vi "SNTP Light RT Driver VI.vi"(6 "Device Clock":string, 9 "Device Inputs FIFO":refnum<k33>, 10 "Device Outputs FIFO":refnum<k33>, 11 "Device Reference":T1 format="%.0x") -> ()   [LabVIEW 2013, in "SNTP Light Custom Device Engine.lvlib"]
uses:
  SNTP Light Custom Device Engine.lvlib
  <vilib>/NI Veristand/Custom Device API/Custom Device Item Ref.ctl
  <vilib>/NI Veristand/Custom Device API/Custom Device Channel Type.ctl
  RT_Configuration_Data.ctl
  <vilib>/NI Veristand/Custom Device API/Custom Device Timed Loop Priority.ctl
  <vilib>/Platform/TimedLoop/XDataNode/timing_clust.ctl
  <vilib>/Platform/TimedLoop/XDataNode/nitl_modes.ctl
  <vilib>/Platform/TimedLoop/XDataNode/wakeup.ctl
  <userlib>/_OpenG.lib/error/error.llb/Filter Error Codes (Array)__ogtk.vi
  <vilib>/NI Veristand/Custom Device API/Get Item Property (String).vi
  <vilib>/NI Veristand/Custom Device API/Get Item Property (U16).vi
  <vilib>/NI Veristand/Custom Device API/Get Item Property (Double).vi
  <vilib>/NI Veristand/Custom Device API/Get Item Property (Boolean).vi
  RT Driver_Global.vi
  <vilib>/platform/TimedLoop/XDataNode/XDataNode.xnode
  <vilib>/NI Veristand/Custom Device API/Custom Device API.lvlib
  <vilib>/NI Veristand/Custom Device Tools/Custom Device Utility Library/Custom Device Utility Library.lvlib
  <vilib>/NI_Real-Time Target Support.lvlib
  <vilib>/nisyscfg/nisyscfg.lvlib
  <vilib>/Platform/TimedLoop/XDataNode/XDNodeRunTimeDep.lvlib
panel:
  in  "stop":bool
  in  "Initialization Status Notifier":refnum<notifier>
  in  "Status Notifier":refnum<notifier>
  # "Custom Device Template\nv1.0"
  # "Use this template as a starting point for creating a custom device code module. The input controls shown here are specially named controls that the system will use to provide the device loop with data. The controls are not required for the device loop to run. For instance, if the device doesn't produce any output data, then you don't need the Device Outputs FIFO control. If you do use these controls, however, they need to have these exact names to be functional."
  # "The optional status notifier element is used to notify the RT engine of the last state of the custom device, and to indicate the device has completed execution. If this control is not used, a default No Error value is returned to the system when the device finishes execution.\n\nNote: This error state is not checked until the system shuts down. Use an output status channel to send more immediate status values to the system."
  # "This optional input can be used to send the VeriStand Engine the final status of the custom device initalization process. If this control exists on the custom device front panel, the VeriStand Engine will wait for a status update before starting up. If the custom device reports an error, that will abort the execution of the current configuration in the VeriStand Engine.\n\nThis control can be deleted if the custom device does not need to send the initialization status update."
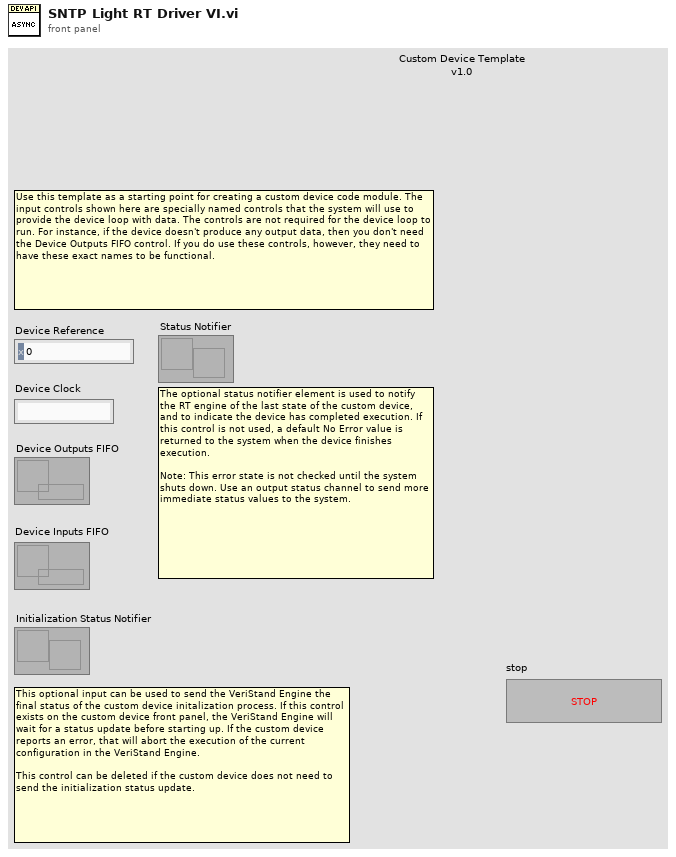
[diagram p1: front panel]
types:
  T1 = typedef "Custom Device API.lvlib/Custom Device Item Ref.ctl" = u64
  T2 = typedef "SNTP Light Custom Device Engine.lvlib/RT_Configuration_Data.ctl" = cluster{"Server IP Address":string, "UDP Port":u16, "Synchronization Interval":dbl, "Synchronization Threshold":dbl, "Debug Output Strings":bool, "Maximum Offset To Apply":dbl}
  T3 = typedef "Custom Device API.lvlib/Custom Device Channel Type.ctl" = enum16{"Input", "Output"}
  T4 = typedef "Custom Device API.lvlib/Custom Device Timed Loop Priority.ctl" = enum32{"Low", "Medium", "High"}
  T5 = typedef "XDNodeRunTimeDep.lvlib/timing_clust.ctl" = cluster{"Expected End [f-1]":u64, "Actual End [f-1]":u64, "Finished Late? [f-1]":bool, "Expected End [i-1]":u64, "Actual End [i-1]":u64, "Finished Late? [i-1]":bool, "Expected Start [i]":u64, "Actual Start [i]":u64, "Expected Start [f]":u64, "Actual Start [f]":u64, "Source Name":string, "Structure Name":string, "Period":i64, "Deadline":i64, "Offset":i64, "Start":i64, "Priority":i32, "Timeout":i32, "Mode":T6, "Wakeup Reason":T7, "Error":errorcluster, "Source Type":string, "Secondary Source Type":string, "Global End Time":u64, "Global Start Time":u64, "Frame Duration":u64, "Iteration Duration":u64, "Assigned CPU":i32, "I/O Scan Engine Mode":u32}
  T6 = typedef "XDNodeRunTimeDep.lvlib/nitl_modes.ctl" = enum32{"No Change", "Process missed periods, maintain original phase", "Discard missed periods, maintain original phase", "Process missed periods, ignore original phase", "Discard missed periods, ignore original phase"}
  T7 = typedef "XDNodeRunTimeDep.lvlib/wakeup.ctl" = enum32{"Normal", "Aborted", "Asynchronous wakeup", "Timing source error", "Timed loop error", "Timeout"}
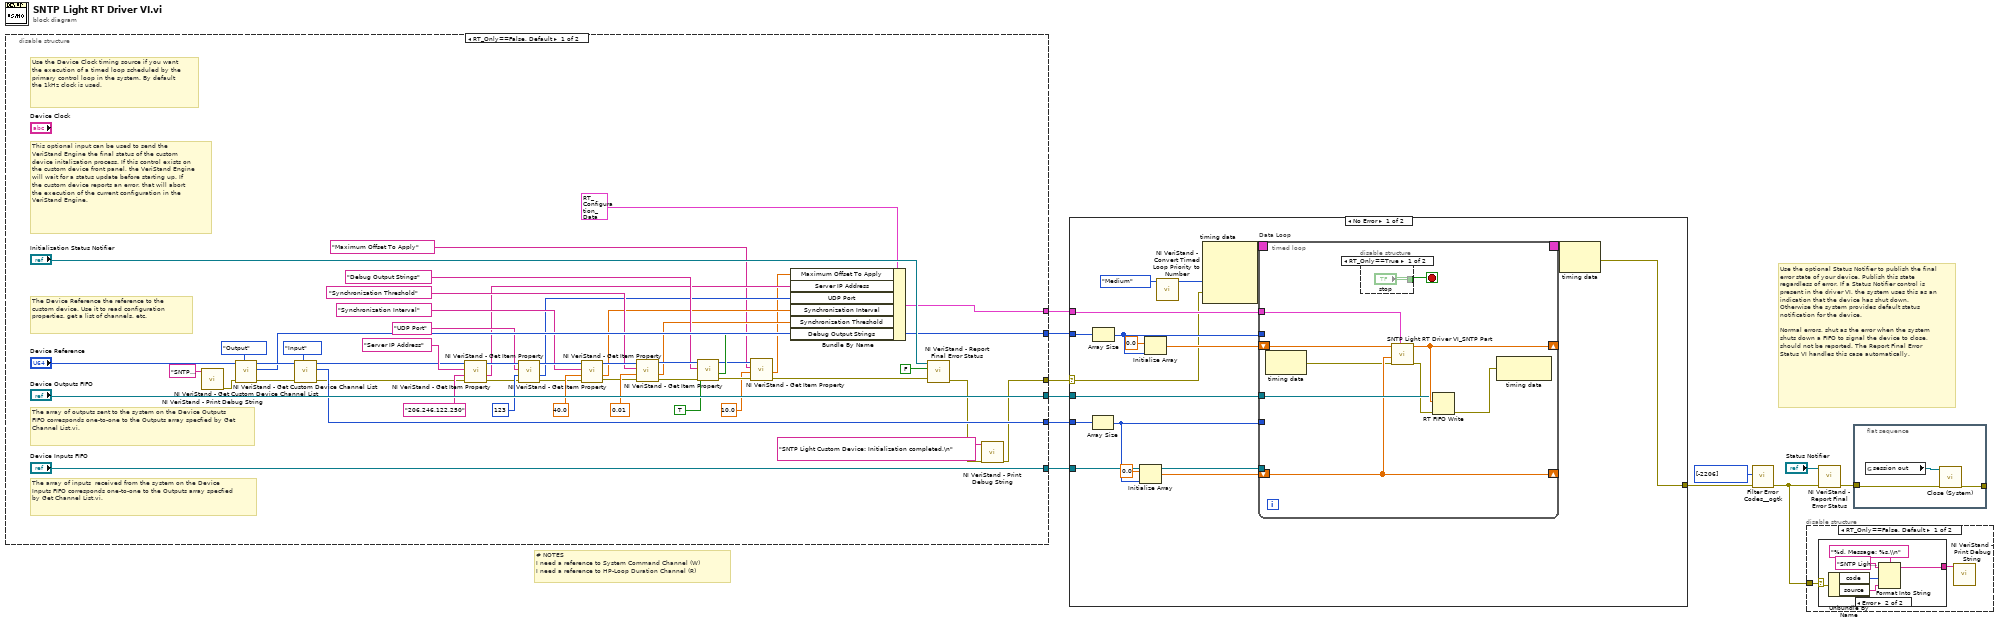
[diagram p0: block diagram]
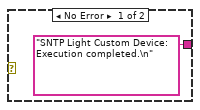
[diagram p2: hidden frame]
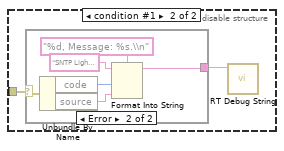
[diagram p3: hidden frame]
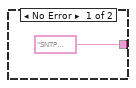
[diagram p4: hidden frame]
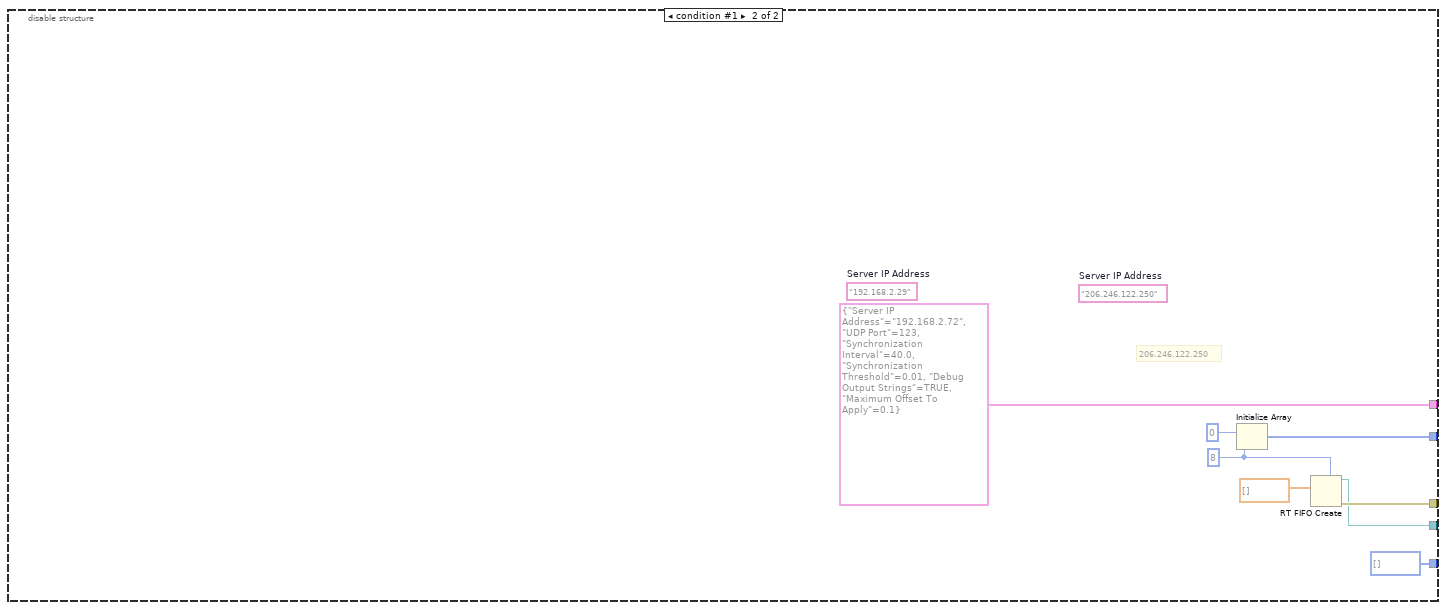
[diagram p5: hidden frame]
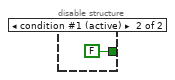
[diagram p6: hidden frame]
diagram:
  # "# NOTES\nI need a reference to System Command Channel (W)\nI need a reference to HP-Loop Duration Channel (R)"
  # "Use the optional Status Notifier to publish the final error state of your device. Publish this state regardless of error. If a Status Notifier control is present in the driver VI, the system uses this as an indication that the device has shut down. Otherwise the system provides default status notification for the device.\n\nNormal errors, shut as the error when the system shuts down a FIFO to signal the device to close, should not be reported. The Report Final Error Status VI handles this case automatically."
  n1 = disable-structure shown="RT_Only==False, Default" {
    disable-tunnel: ["Device Outputs FIFO" w63] -> w11
    disable-tunnel: ["Device Inputs FIFO" _] -> w10
    disable-tunnel: [w53 T1[] [] ("Specified Channel Ref List")] -> w9
    disable-tunnel: [w52 w65] -> w8
    disable-tunnel: [w21 w64] -> w6
    disable-tunnel: [w23 T2 {"Server IP Address"="192.168.2.72", "UDP Port"=123, "Synchronization Interval"=40.0, "Synchronization Threshold"=0.01, "Debug Output Strings"=TRUE, "Maximum Offset To Apply"=0.1} ("Configuration")] -> w5
    frame condition #0 (active) {
      # "This optional input can be used to send the VeriStand Engine the final status of the custom device initalization process. If this control exists on the custom device front panel, the VeriStand Engine will wait for a status update before starting up. If the custom device reports an error, that will abort the execution of the current configuration in the VeriStand Engine."
      # "The array of inputs  received from the system on the Device Inputs FIFO corresponds one-to-one to the Outputs array specfied by Get Channel List.vi."
      # "The array of outputs sent to the system on the Device Outputs FIFO corresponds one-to-one to the Outputs array specfied by Get Channel List.vi."
      # "The Device Reference the reference to the custom device. Use it to read configuration properties, get a list of channels, etc."
      # "Use the Device Clock timing source if you want the execution of a timed loop scheduled by the primary control loop in the system. By default the 1kHz clock is used."
      n2 = call <vilib>:"NI VeriStand - Print Debug String.vi"("Message"="SNTP Light Custom Device: Initialization started.\n") -> ("error out"=w18:errorcluster)  [unwired: 10 in]
      n3 = call <vilib>:"NI VeriStand - Get Custom Device Channel List.vi"("Channel Type"=Custom_Device_Channel_Type."Output", "error in (no error)"=w18, "Device Ref in"="Device Reference") -> ("error out"=w55:errorcluster, "Specified Channel Ref List"=w52:T1[], "Device Ref out"=w56:T1)  [unwired: 6 out]
      n4 = call <vilib>:"NI VeriStand - Get Custom Device Channel List.vi"("Channel Type"=Custom_Device_Channel_Type."Input", "error in (no error)"=w55, "Device Ref in"=w56) -> ("error out"=w30:errorcluster, "Specified Channel Ref List"=w53:T1[], "Device Ref out"=w31:T1)  [unwired: 6 out]
      n5 = call-poly <vilib>:"NI VeriStand - Get Item Property.vi"("error in (no error)"=w30, "Default Value"="206.246.122.250" ("Value"), "Property Name"="Server IP Address", "Item Ref in"=w31) -> ("error out"=w43:errorcluster, "Value"=w28:string, "Item Ref out"=w45:T1)  [unwired: 4 in, 1 out]
      n6 = call-poly <vilib>:"NI VeriStand - Get Item Property.vi"("error in (no error)"=w43, "Default Value"=u16 123 ("Value"), "Property Name"="UDP Port", "Item Ref in"=w45) -> ("error out"=w42:errorcluster, "Value"=w27:u16, "Item Ref out"=w44:T1)  [unwired: 4 in, 1 out]
      n7 = call-poly <vilib>:"NI VeriStand - Get Item Property.vi"("error in (no error)"=w42, "Default Value"=40.0 ("Value"), "Property Name"="Synchronization Interval", "Item Ref in"=w44) -> ("error out"=w37:errorcluster, "Value"=w26:dbl, "Item Ref out"=w38:T1)  [unwired: 4 in, 1 out]
      n8 = call-poly <vilib>:"NI VeriStand - Get Item Property.vi"("error in (no error)"=w37, "Default Value"=0.01 ("Value"), "Property Name"="Synchronization Threshold", "Item Ref in"=w38) -> ("error out"=w34:errorcluster, "Value"=w25:dbl, "Item Ref out"=w35:T1)  [unwired: 4 in, 1 out]
      n9 = call-poly <vilib>:"NI VeriStand - Get Item Property.vi"("error in (no error)"=w34, "Default Value"=TRUE ("Value"), "Property Name"="Debug Output Strings", "Item Ref in"=w35) -> ("error out"=w15:errorcluster, "Value"=w24:bool, "Item Ref out"=w17:T1)  [unwired: 4 in, 1 out]
      n10 = call-poly <vilib>:"NI VeriStand - Get Item Property.vi"("error in (no error)"=w15, "Default Value"=10.0, "Property Name"="Maximum Offset To Apply", "Item Ref in"=w17) -> ("error out"=w16:errorcluster, "Value"=w13:dbl)  [unwired: 4 in, 2 out]
      n11 = Bundle By Name(cluster=T2 {"Server IP Address"="206.246.122.250", "UDP Port"=123, "Synchronization Interval"=60.0, "Synchronization Threshold"=0.01, "Debug Output Strings"=TRUE, "Maximum Offset To Apply"=0.0} ("Configuration"), "Maximum Offset To Apply"=w13, "Server IP Address"=w28, "UDP Port"=w27, "Synchronization Interval"=w26, "Synchronization Threshold"=w25, "Debug Output Strings"=w24) -> (w23:T2)
      n12 = call <vilib>:"NI VeriStand - Report Final Error Status.vi"("error in (no error)"=w16, "Filter FIFO & Shutdown Errors (T)"=FALSE ("Filter FIFO Errors (T)"), "Status Notifier"="Initialization Status Notifier") -> ("error out"=w22:errorcluster)  [unwired: 8 out]
      n13 = call <vilib>:"NI VeriStand - Print Debug String.vi"("error in (no error)"=w22, "Message"="SNTP Light Custom Device: Initialization completed.\n") -> ("error out"=w21:errorcluster)  [unwired: 9 in]
    }
    frame condition #1 {
      (unwired) "206.246.122.250"  # Server IP Address
      (unwired) "192.168.2.29"  # Server IP Address
      w62 = 8 ("dimension size")
      # "206.246.122.250"
      n14 = Initialize Array(T1 0 ("Device Item Ref"), w62) -> (w65:T1[])
      n15 = RT FIFO Create(1:dbl[] [], 6:w62) -> (8:w63:refnum<k33>, 11:w64:errorcluster)  [unwired: 6 in, 1 out]
    }
  }
  n16 = case shown="No Error" w6 {
    selector: w6 -> [w72 w108]
    tunnel: w11 -> [w85 _]
    tunnel: w10 -> [w84 _]
    tunnel: w9 -> [w78 _]
    tunnel: w8 -> [w77 _]
    tunnel: [w69 w108] -> w3
    tunnel: w5 -> [w75 _]
    frame No Error {
      n17 = Array Size(array=w78) -> (size(s)=w76:i32)
      n18 = Array Size(array=w77) -> (size(s)=w79:i32)
      n19 = Initialize Array(0.0 ("element"), w76) -> (w80:dbl[])
      n20 = Initialize Array(0.0 ("element"), w79) -> (w81:dbl[])
      n21 = call <vilib>:"NI VeriStand - Convert Timed Loop Priority to Number.vi"("Priority"=Custom_Device_Timed_Loop_Priority."Medium") -> ("Numeric Priority"=w70:i32)  [unwired: 10 in]
      n22 = node-c288(w70, w72) -> (w74:T5)  [unwired: 2 in]
      n23 = timed-loop "Data Loop" {
        shift-right: [w87] -> _
        shift-left: w80 -> [w87]
        shift-right: [w93] -> _
        shift-left: w81 -> [w94]
        tunnel: w79 -> [_]
        tunnel: w85 -> [w92]
        tunnel: w84 -> [_]
        tunnel: w76 -> [_]
        tunnel: w75 -> [w90]
        timing: w74 -> [_]
        timing-out: [_] -> w73
        stop <- w88 stop-if-true
        n24 = node-c288() -> (w86:errorcluster)  [unwired: 1 in]
        n25 = disable-structure shown="RT_Only==True" {
          disable-tunnel: ["stop" FALSE ("stop")] -> w88
          frame condition #0 {
          }
          frame condition #1 (active) {
          }
        }
        n26 = call "SNTP Light RT Driver VI_SNTP Part.vi"("Configuration"=w90, "error in (no error)"=w86, "Inputs In"=w87, "Outputs In"=w94) -> ("error out"=w91:errorcluster, "Outputs Out"=w93:dbl[])  [unwired: 6 in]
        n27 = RT FIFO Write(0:w92, 1:w93, 3:w91) -> (11:w89:errorcluster)  [unwired: 1 in, 4 out]
        n28 = node-c288(w89) -> ()  [unwired: 1 out]
      }
      n29 = node-c288(w73) -> (w69:errorcluster)
    }
    frame Error {
    }
  }
  n30 = call-poly <userlib>:"Filter Error Codes__ogtk.vi"("Error In"=w3, "Error Codes to Filter"=i32[] [-2206]) -> ("Error Out"=w1:errorcluster)  [unwired: 7 in, 2 out]
  n31 = disable-structure shown="RT_Only==False, Default" {
    disable-tunnel: w1 -> [w109 w119]
    frame condition #0 (active) {
      n32 = case shown="Error" w109 {
        selector: w109 -> [_ w117]
        tunnel: ["SNTP Light Custom Device: Execution completed.\n" ("Message") w112] -> w110
        frame No Error {
        }
        frame Error {
          n33 = Unbundle By Name(w117) -> ("code"=w116:i32, "source"=w115:string)
          n34 = Format Into String(format string="%d, Message: %s.\\n", initial string="SNTP Light Custom Device: Execution completed with error: Code: " ("Message"), w116, w115) -> (resulting string=w112:string)  [unwired: 1 in, 1 out]
        }
      }
      n35 = call <vilib>:"NI VeriStand - Print Debug String.vi"("Message"=w110) -> ()  [unwired: 10 in, 1 out]
    }
    frame condition #1 {
      n36 = case shown="Error" w119 {
        selector: w119 -> [_ w126]
        tunnel: ["SNTP Light Custom Device: Execution completed.\n" ("Message") w121] -> w118
        frame No Error {
        }
        frame Error {
          n37 = Unbundle By Name(w126) -> ("code"=w125:i32, "source"=w124:string)
          n38 = Format Into String(format string="%d, Message: %s.\\n", initial string="SNTP Light Custom Device: Execution completed with error: Code: " ("Message"), w125, w124) -> (resulting string=w121:string)  [unwired: 1 in, 1 out]
        }
      }
      n39 = call <vilib>:"RT Debug String.vi"("String to write"=w118) -> ()  [unwired: 10 in, 1 out]
    }
  }
  n40 = call <vilib>:"NI VeriStand - Report Final Error Status.vi"("error in (no error)"=w1, "Status Notifier"="Status Notifier") -> ("error out"=w4:errorcluster)  [unwired: 1 in, 8 out]
  n41 = flat-sequence {
    tunnel: w4 -> [w129]
    tunnel: [w128] -> _
    frame #0 {
      n42 = global read "RT Driver_Global.vi" "session out"() -> (w127:refnum<k21>)
      n43 = call <vilib>:"Close (System).vi"("error in (no error)"=w129, "session in"=w127) -> ("error out"=w128:errorcluster)  [unwired: 9 in]
    }
  }
